vi "Test 8.vi"() -> ()   [LabVIEW 2019]
panel:
  out "In Range?":bool
  in  "Lower [CAD]":fxp<+,18,11>
  in  "Upper [CAD]":fxp<+,18,11>
  in  "Angle [CAD]":fxp<+,18,11>
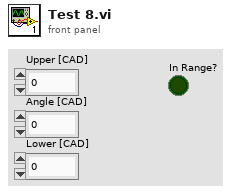
[diagram p1: front panel]
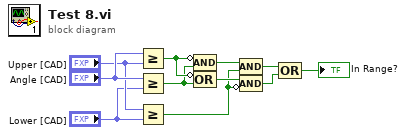
[diagram p0: block diagram]
diagram:
  n1 = Greater Or Equal?(x="Angle [CAD]", y="Upper [CAD]") -> (x >= y?=w5:bool)
  n2 = Greater Or Equal?(x="Angle [CAD]", y="Lower [CAD]") -> (x >= y?=w4:bool)
  n3 = Greater Or Equal?(x="Upper [CAD]", y="Lower [CAD]") -> (x >= y?=w1:bool)
  n4 = Compound Arithmetic op=AND(invert w5, w4) -> (w3:bool)
  n5 = Compound Arithmetic op=OR(invert w5, w4) -> (w7:bool)
  n6 = Compound Arithmetic op=AND(w3, w1) -> (w2:bool)
  n7 = Compound Arithmetic op=AND(w7, invert w1) -> (w6:bool)
  n8 = Compound Arithmetic op=OR(w2, w6) -> (→"In Range?":bool)
